vi "[Point Reactor Simulate].vi"() -> ()   [LabVIEW 2020]
doc: "本程序通过点堆动力学模型模拟核电站的反应堆运行状态。"
uses:
  <vilib>/Instr/_visa.llb/VISA Find Search Mode.ctl
  <vilib>/Utility/sysdir.llb/System Directory Type.ctl
  <vilib>/Utility/error.llb/DialogType.ctl
  Utility/Typedefs/KE622x -- Instrument Type.ctl
  Configure/Source/Typedefs/KE622x -- Voltage Limit.ctl
  Configure/Source/Typedefs/KE622x -- Current Range.ctl
  Configure/Source/Typedefs/KE622x -- Current Ranges.ctl
  <vilib>/DAQmx/write.llb/DAQmx Write (Counter 1D Frequency 1Chan NSamp).vi
  <vilib>/DAQmx/write.llb/DAQmx Write (Analog DBL 1Chan 1Samp).vi
  <vilib>/Analysis/polynomials.llb/Scalar Polynomial Evaluation (DBL).vi
  <vilib>/Instr/_visa.llb/VISA Configure Serial Port (Instr).vi
  <vilib>/DAQmx/create/channels.llb/DAQmx Create Channel (CO-Pulse Generation-Frequency).vi
  <vilib>/DAQmx/configure/timing.llb/DAQmx Timing (Implicit).vi
  <vilib>/DAQmx/create/channels.llb/DAQmx Create Channel (AO-Voltage-Basic).vi
  <vilib>/DAQmx/miscellaneous.llb/DAQmx Fill In Error Info.vi
  TcpModbus_SlaveServer/MB Slave Init (poly).vi
  TcpModbus_SlaveServer/MB Globals.vi
  TcpModbus_SlaveServer/MB Slave Read Holding Registers (poly).vi
  TcpModbus_SlaveServer/MB Slave Write Input Registers (poly).vi
  PointReactorDll.dll
  <vilib>/Analysis/NI_AALPro.lvlib
  Keithley 622x.lvlib
  <resource>/objmgr/daqmx.rc
panel:
  out "KE6220_2":bool
  in  "物理参数设置":bool
  in  "endian Switch":bool
  out "反应性仪输出电压":dbl[](array[numeric])
  out "输出电压":dbl[](array[numeric])
  in  "输出电流 (A)":dbl
  in  "电压输出选择":bool
  out "中子注量率 (n/cm2·s)":dbl
  out "硼总价值 (pcm)":dbl
  out "棒总价值 (pcm)":dbl
  out "硼浓度 indicator":dbl
  in  "硼浓度 (ppm)":dbl(slide)=1.0 scale=0.0..2000.0
  out "运行时间 (s)":dbl
  in  "TCP端口号":u16=502 min=1 max=9999
  out "堆芯反应性(硼+棒) (pcm)":dbl
  out "keff":dbl
  in  "S棒组":dbl(slide)=100.0 min=0.0 max=225.0 scale=0.0..225.0
  in  "A棒组":dbl(slide)=100.0 min=0.0 max=225.0 scale=0.0..225.0
  in  "B棒组":dbl(slide)=100.0 min=0.0 max=225.0 scale=0.0..225.0
  in  "C棒组":dbl(slide)=100.0 min=0.0 max=225.0 scale=0.0..225.0
  in  "堆芯后备反应性 (pcm)":dbl
  out "S棒价值":dbl
  out "A棒价值":dbl
  out "B棒价值":dbl
  out "C棒价值":dbl
  out "D棒价值":dbl
  out "中子注量曲线":dbl(graph) caption="Waveform Chart - Dark"
  in  "D棒组":dbl(slide)=100.0 min=0.0 max=225.0 scale=0.0..225.0
  out "CARD":bool
  out "KE6220_1":bool
  out "COM2":bool
  out "COM1":bool
  in  "VO 4":u16(ring)=3 items=["D棒位 (step)", "C棒位 (step)", "B棒位 (step)", "A棒位 (step)", "S棒位 (step)", "硼浓度 (ppm)", "中间量程电流 (A)", "源量程计数 (CPS)"]
  in  "VO 3":u16(ring)=2 items=["D棒位 (step)", "C棒位 (step)", "B棒位 (step)", "A棒位 (step)", "S棒位 (step)", "硼浓度 (ppm)", "中间量程电流 (A)", "源量程计数 (CPS)"]
  in  "VO 2":u16(ring)=1 items=["D棒位 (step)", "C棒位 (step)", "B棒位 (step)", "A棒位 (step)", "S棒位 (step)", "硼浓度 (ppm)", "中间量程电流 (A)", "源量程计数 (CPS)"]
  in  "VO 1":u16(ring) items=["D棒位 (step)", "C棒位 (step)", "B棒位 (step)", "A棒位 (step)", "S棒位 (step)", "硼浓度 (ppm)", "中间量程电流 (A)", "源量程计数 (CPS)"]
  in  "电信号输出设置":bool
  in  "TCP服务器开":bool
  out "Holding Registers":sgl[](array[numeric]) caption="Holding Registers (Read&Write)"
  out "Coils":bool[](array[boolean]) caption="Coils (Master can write coils)"
  in  "电流输出选择":u16(ring) items=["中间量程电流", "功率量程电流"]
  out "棒位与硼浓度":dbl[](array[numeric])
  in  "反应性控制方式":bool
  in  "归零":bool
  in  "棒速(step/min)":dbl=72.0 min=1.0 max=10000.0 step=1.0 format="%#.3g"
  in  "开始降棒":bool
  in  "降棒选择":u16(ring) items=["D棒组", "C棒组", "B棒组", "A棒组", "S棒组"]
  in  "细分时间 (ms)":u32=100 min=10 max=1000 step=1
  in  "开始":bool
  in  "时间比例尺":dbl(knob)=1.0 min=0.1 max=1000.0 step=0.1 scale=0.1..1000.0
  out "功率量程 (A)":dbl(slide) scale=2.875e-12..0.00023 scale format="%#_6e"
  out "中间量程 (A)":dbl(slide) scale=1e-11..0.0008 scale format="%#_6e"
  out "源量程 (CPS)":dbl(slide) scale=1.0..1000000.0 scale format="%#_6f"
  out "%FP":dbl(slide) scale=2e-09..200.0 scale format="%#_6e"
  out "中子注量率":dbl(slide) scale=0.1..10000000000.0 scale format="%#_6e"
  in  "时间步长 (s)":dbl=0.1
  in  "初始注量率 (n/cm2·s)":dbl=1.0
  in  "堆芯反应性 (pcm)":dbl
  in  "停止":bool
  in  "初始反应性 (pcm)":dbl
  # "反应性仪测试用点堆模拟器"
  # "探测器"
  # "手输"
  # "棒硼"
  # "1.25E+5 n/cm2·s\n——"
  # "——\n1.25E+2 n/cm2·s"
  # "——  1.25E-1 n/cm2·s"
  # "硬件测试"
  # "小端"
  # "0-10V"
  # "1-5V"
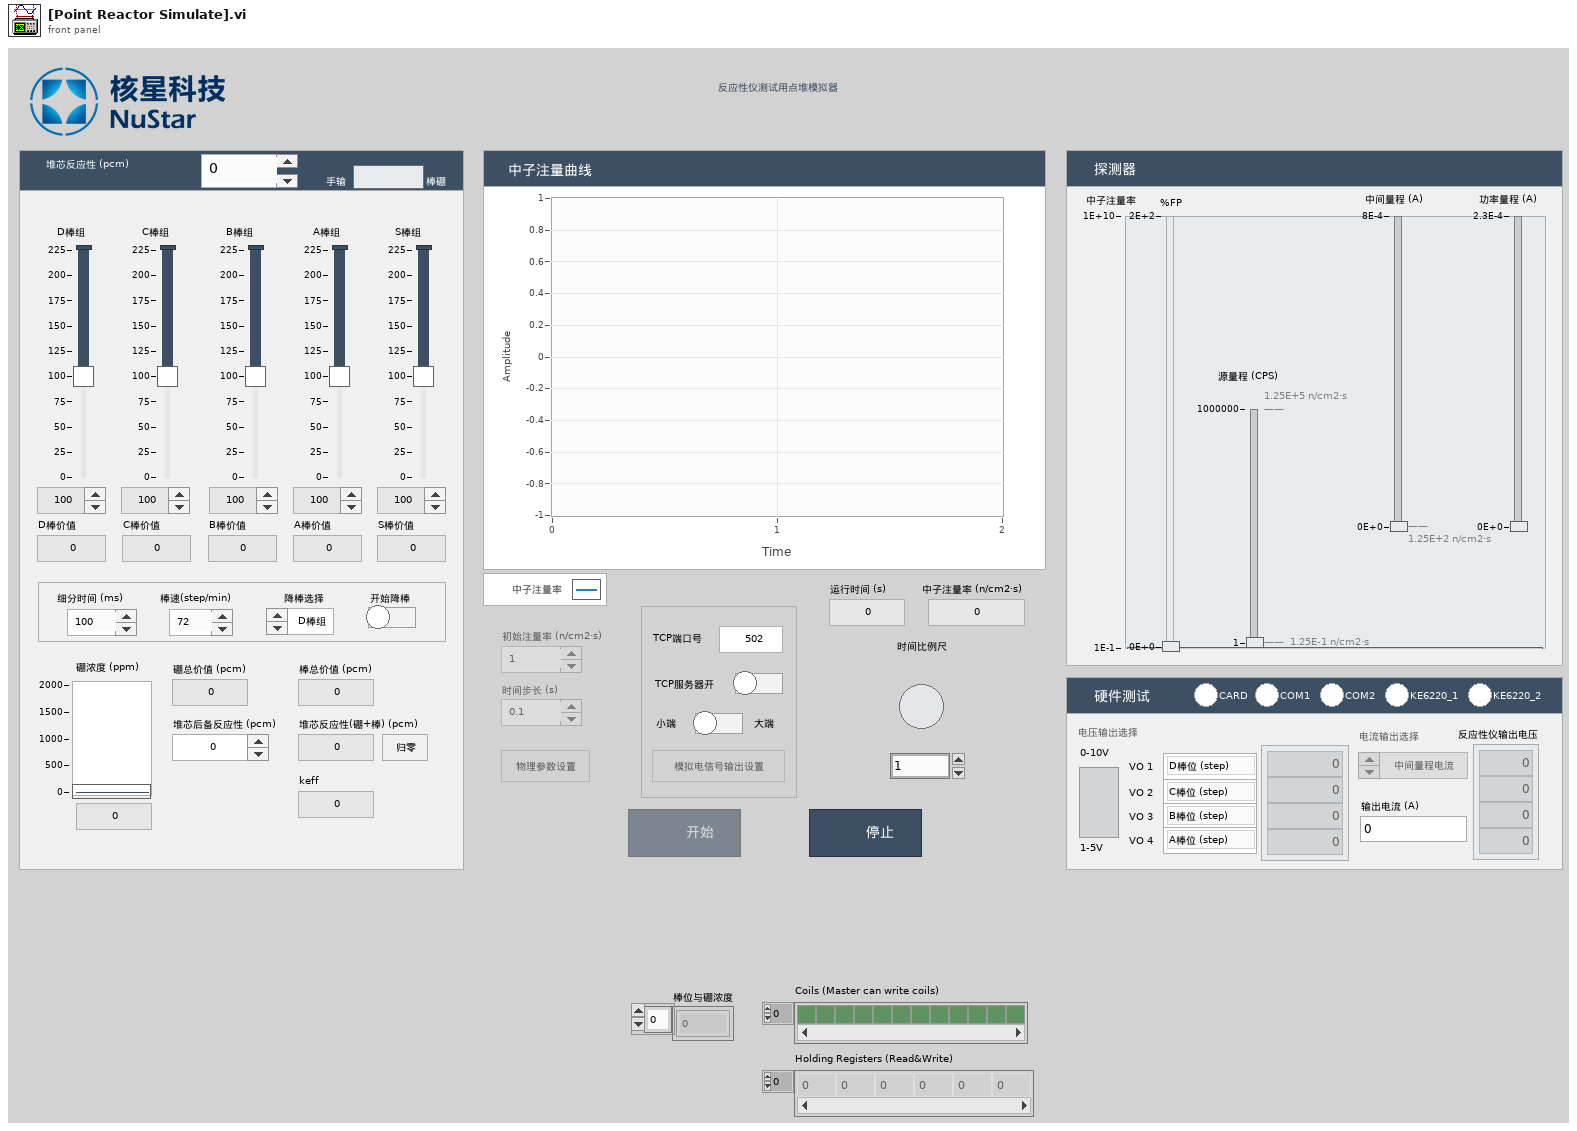
[diagram p1: front panel]
types:
  T1 = enum8{"Enabled", "Disabled", "Disabled and Grayed Out"}
  T2 = typedef "System Directory Type.ctl" = i32
  T3 = typedef "VISA Find Search Mode.ctl" = u32
  T4 = enum16{"open", "open or create", "create or replace", "create", "open (read only)"}
  T5 = typedef "DialogType.ctl" = u16
  T6 = typedef "Keithley 622x.lvlib/KE622x -- Voltage Limit.ctl" = dbl
  T7 = typedef "Keithley 622x.lvlib/KE622x -- Instrument Type.ctl" = enum16{"KE6220", "KE6221"}
  T8 = typedef "Keithley 622x.lvlib/KE622x -- Current Range.ctl" = cluster{"Auto Range?":bool, "Man / Selected\nRange":T9}
  T9 = typedef "Keithley 622x.lvlib/KE622x -- Current Ranges.ctl" = enum16{"2nA", "20nA", "200nA", "2uA", "20uA", "200uA", "2mA", "20mA", "100mA"}
  T10 = enum32{"invalid app kind", "Development System", "Run Time System", "Student Edition", "Embedded LabVIEW", "Evaluation", "Custom"}
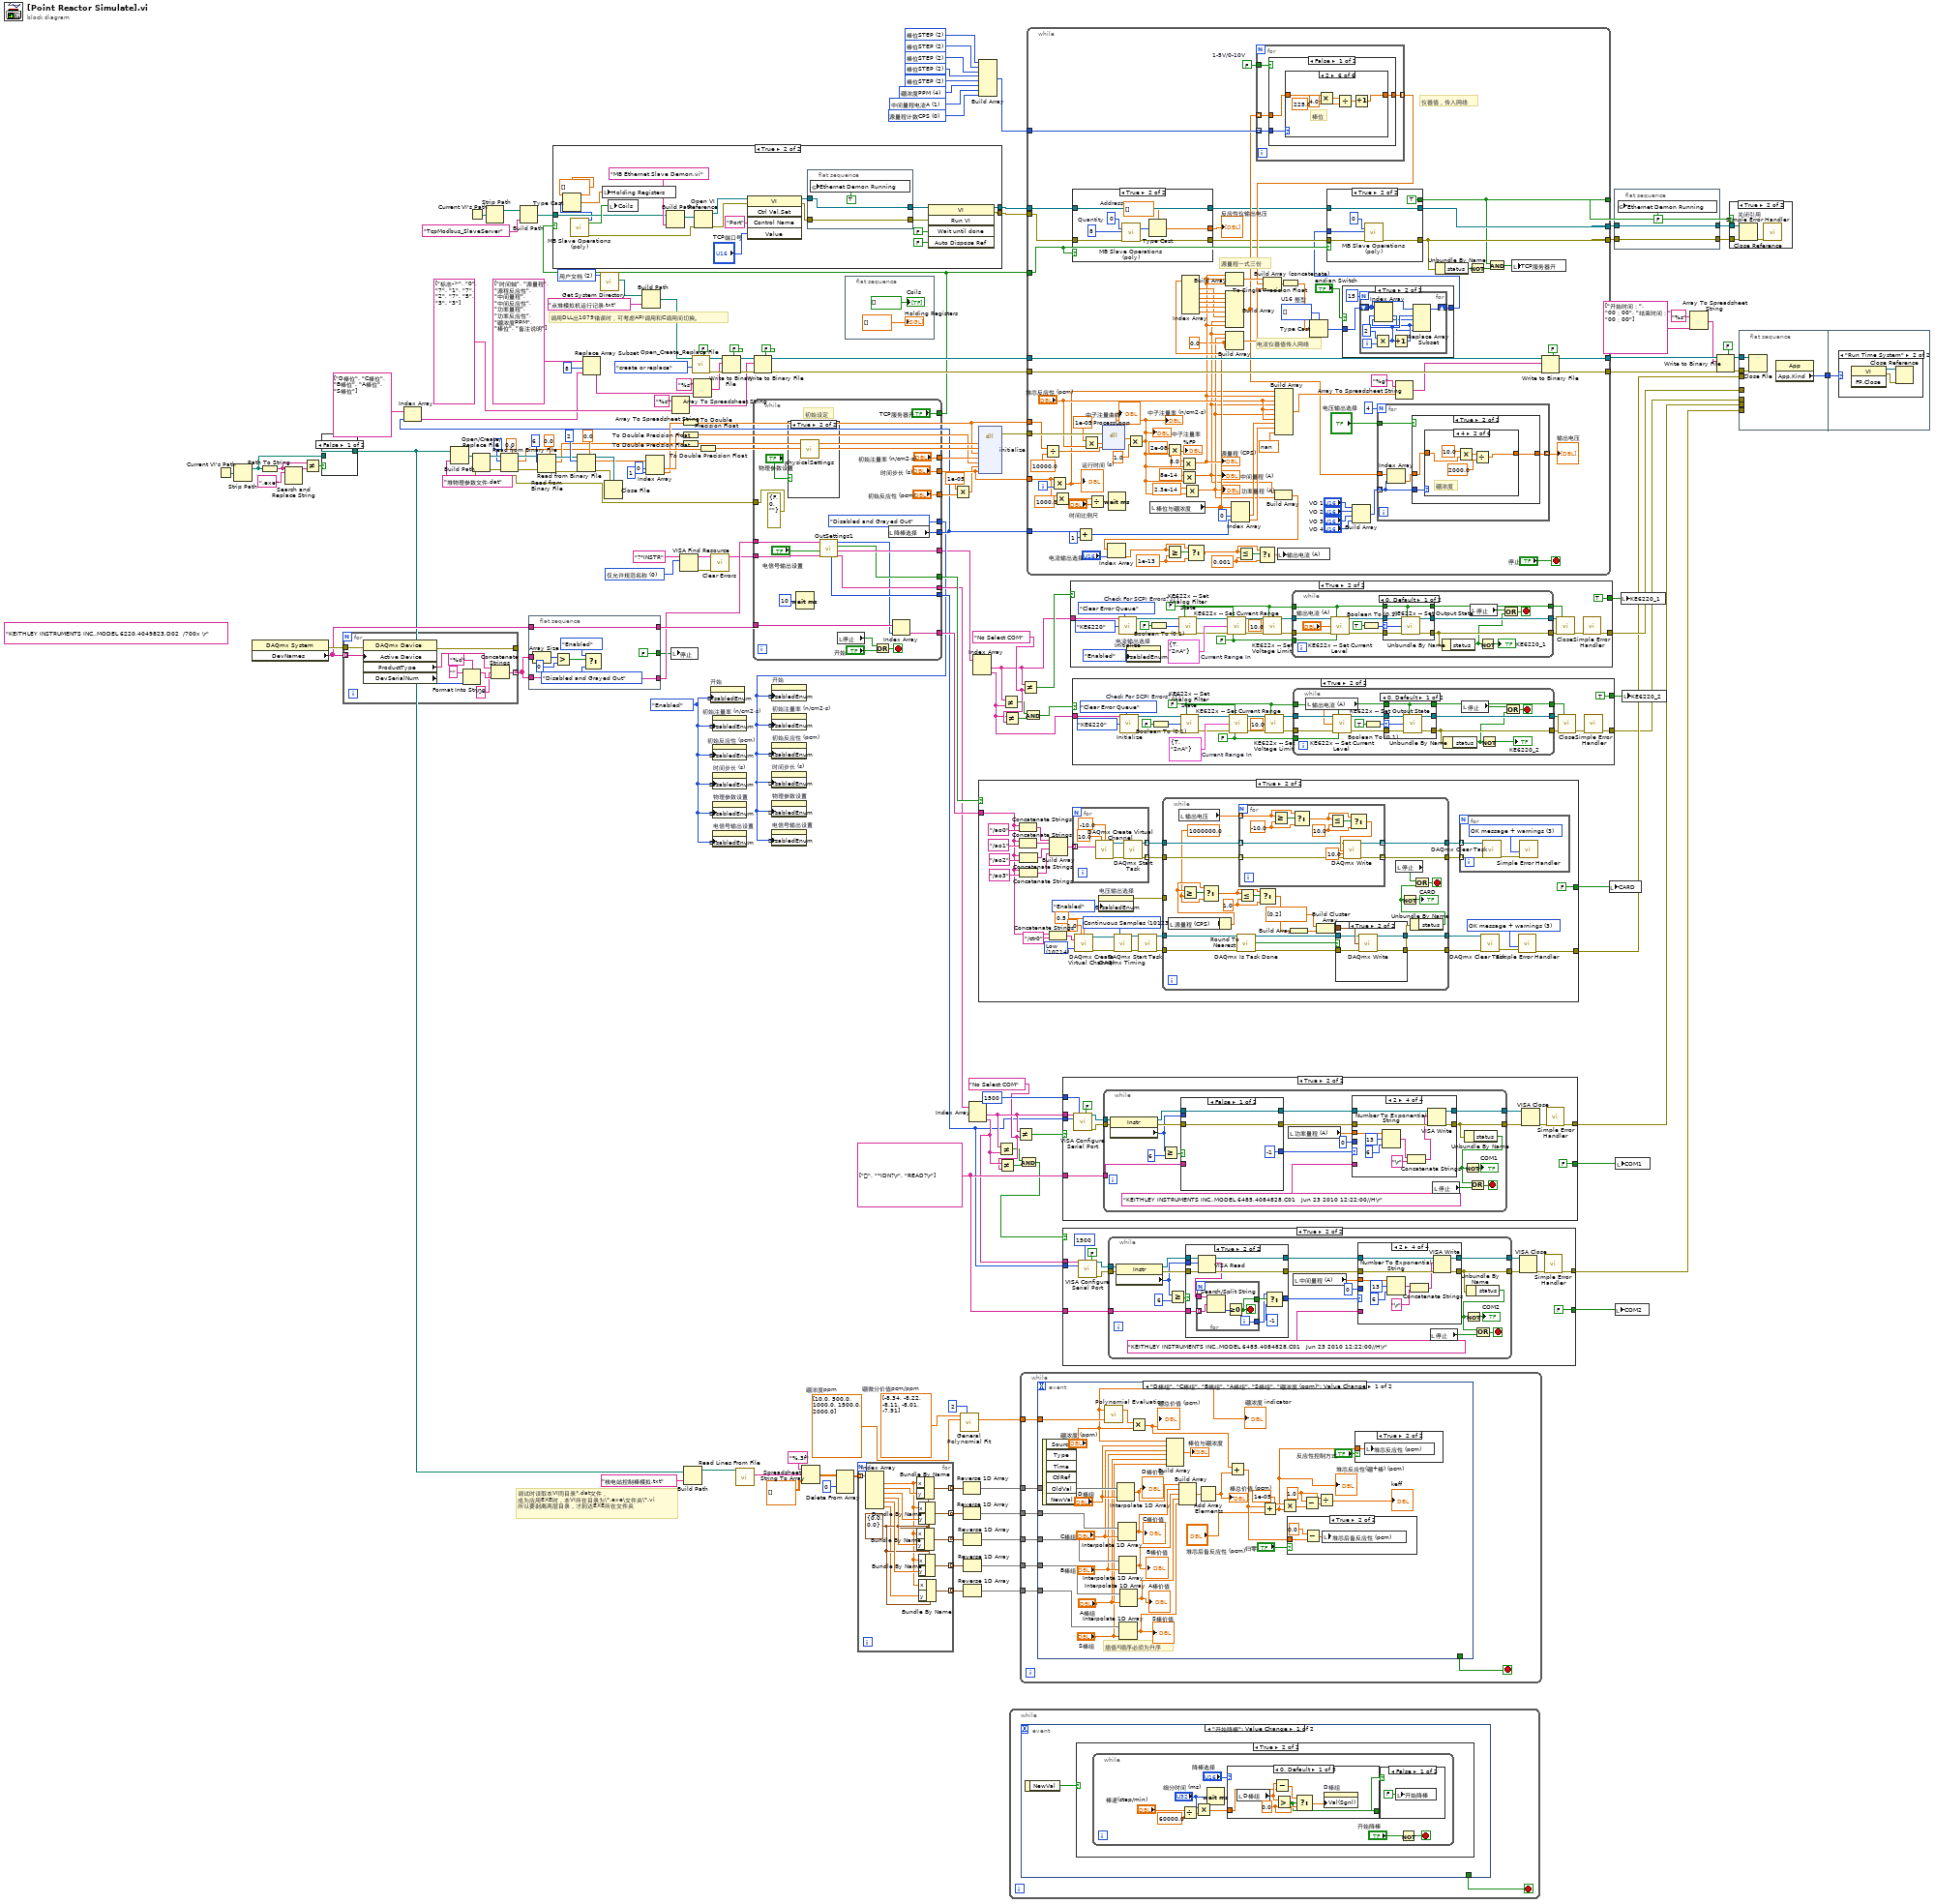
[diagram p0: block diagram]
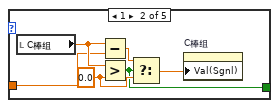
[diagram p4: hidden frame]
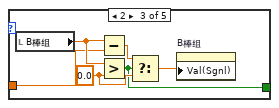
[diagram p5: hidden frame]
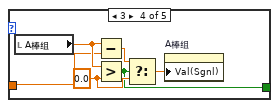
[diagram p6: hidden frame]
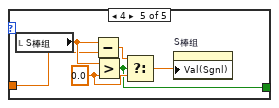
[diagram p7: hidden frame]
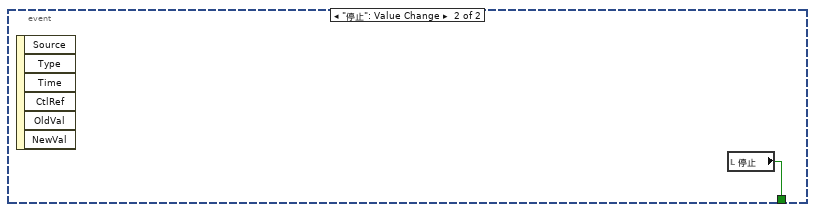
[diagram p8: hidden frame]
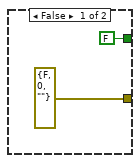
[diagram p9: hidden frame]
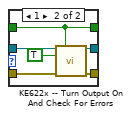
[diagram p10: hidden frame]
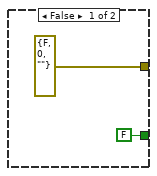
[diagram p11: hidden frame]
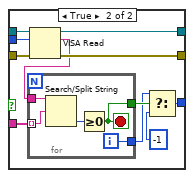
[diagram p12: hidden frame]
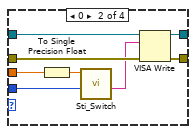
[diagram p14: hidden frame]
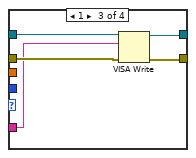
[diagram p15: hidden frame]
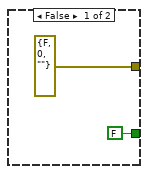
[diagram p16: hidden frame]
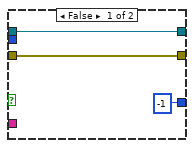
[diagram p17: hidden frame]
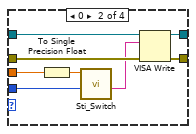
[diagram p19: hidden frame]
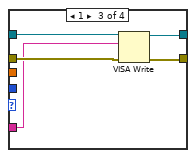
[diagram p20: hidden frame]
diagram:
  w2 = T1."Enabled" ("禁用")
  w10 = "No Select COM" ("新元素/子数组")
  (unwired) "KEITHLEY INSTRUMENTS INC.,MODEL 6220,4049823,D02  /700x \r" ("y")
  w16 = T2 2 items=["用户目录"=0, "用户桌面"=1, "用户文档"=2, "用户应用程序数据"=3, "用户设置"=4, "用户临时目录"=5, "公共文档"=6, "公共应用程序数据"=7, "公共设置"=8, "公共缓存"=13, "系统核心库"=9, "系统安装库"=10, "应用程序文件"=11, "启动盘根目录"=12] ("system directory type")
  w36 = "No Select COM" ("新元素/子数组")
  w41 = string[] ["", "*IDN?\r", "READ?\r"] ("添加的数组")
  w51 = u16 0 items=["源量程计数CPS", "中间量程电流A", "棒位STEP", "温度(摄氏度)", "硼浓度PPM", "P2电压信号"] ("P2-8")
  w50 = u16 1 items=["源量程计数CPS", "中间量程电流A", "棒位STEP", "温度(摄氏度)", "硼浓度PPM", "P2电压信号"] ("P2-7")
  w49 = u16 4 items=["源量程计数CPS", "中间量程电流A", "棒位STEP", "温度(摄氏度)", "硼浓度PPM", "P2电压信号"] ("P2-6")
  w48 = u16 2 items=["源量程计数CPS", "中间量程电流A", "棒位STEP", "温度(摄氏度)", "硼浓度PPM", "P2电压信号"] ("P2-5")
  w47 = u16 2 items=["源量程计数CPS", "中间量程电流A", "棒位STEP", "温度(摄氏度)", "硼浓度PPM", "P2电压信号"] ("P2-4")
  w46 = u16 2 items=["源量程计数CPS", "中间量程电流A", "棒位STEP", "温度(摄氏度)", "硼浓度PPM", "P2电压信号"] ("P2-3")
  w45 = u16 2 items=["源量程计数CPS", "中间量程电流A", "棒位STEP", "温度(摄氏度)", "硼浓度PPM", "P2电压信号"] ("P2-2")
  w44 = u16 2 items=["源量程计数CPS", "中间量程电流A", "棒位STEP", "温度(摄氏度)", "硼浓度PPM", "P2电压信号"] ("P2-1")
  w64 = T3 0 items=["仅允许规范名称"=0, "只允许别名"=2, "包含匹配别名"=3, "包含所有别名"=4] ("Search Mode")
  w90 = dbl[] [-8.34, -8.22, -8.11, -8.01, -7.91]  # 硼微分价值pcm/ppm
  w89 = dbl[] [10.0, 500.0, 1000.0, 1500.0, 2000.0]  # 硼浓度ppm
  # "调试时读取本VI同目录*.dat文件，\n成为应用EXE时，本VI所在目录为\\*.exe\\文件夹\\*.vi\n所以要剥离两层目录，才到达EXE所在文件夹"
  # "调用DLL出1079错误时，可考虑API调用和C调用间切换。"
  n1 = Current VI's Path() -> (path=w124:path)
  n2 = Strip Path(path=w124) -> (stripped path=w119:path)  [unwired: 1 out]
  n3 = property class="DAQmx System"() -> (error out=w70:errorcluster, "DevNames"=w68:tag[])  [unwired: 2 in, 1 out]
  n4 = Path To String(path=w119) -> (string=w121:string)
  n5 = Search and Replace String(input string=w121, search string=".exe" ("搜索字符串")) -> (result string=w122:string)  [unwired: 6 in, 3 out]
  n6 = Not Equal?(x=w121, y=w122) -> (x != y?=w120:bool)
  n7 = case shown="False" w120 {
    tunnel: w119 -> [w162 w164]
    tunnel: [w162 w163] -> w18
    frame False {
    }
    frame True {
      n8 = Strip Path(path=w164) -> (stripped path=w163:path)  [unwired: 1 out]
    }
  }
  n9 = for {
    tunnel: w68 -> [w174] mode=indexing
    tunnel: w70 -> [w173]
    tunnel: [w172] -> _
    tunnel: [w165] -> w69 mode=indexing
    n10 = property class="DAQmx Device"(error in=w173, "Active Device"=w174) -> (error out=w172:errorcluster, "ProductType"=w168:string, "DevSerialNum"=w169:u32)  [unwired: 1 in, 1 out]
    n11 = Format Into String(format string="%d" ("格式字符串"), initial string="" ("初始字符串"), w169) -> (resulting string=w167:string)  [unwired: 1 in, 1 out]
    n12 = Concatenate Strings(w168, "-" ("字符串"), w167) -> (w165:string)
  }
  n13 = Build Path(base path=w18, name or relative path="堆物理参数文件.dat") -> (appended path=w125:path)
  n14 = Current VI's Path() -> (path=w56:path)
  n15 = Strip Path(path=w56) -> (stripped path=w55:path)  [unwired: 1 out]
  n16 = Build Path ("创建路径")(base path=w55, name or relative path="TcpModbus_SlaveServer" ("搜索字符串")) -> (appended path=w54:path)
  n17 = flat-sequence {
    tunnel: w69 -> [w183]
    tunnel: [w178] -> w42
    tunnel: w69 -> [w178]
    tunnel: w68 -> [w177]
    tunnel: [w177] -> w67
    tunnel: [FALSE ("停止")] -> w27
    frame #0 {
      n18 = Array Size(array=w183) -> (size(s)=w182:i32)
      n19 = Greater?(x=w182, y=0) -> (0:w179:bool)
      n20 = Select(t=T1."Enabled" ("禁用"), s=w179, f=T1."Disabled and Grayed Out" ("禁用")) -> ()  [unwired: 1 out]
    }
  }
  n21 = call <vilib>:"Get System Directory.vi"("system directory type"=w16) -> ("system directory"=w17:path)  [unwired: 10 in]
  n22 = Build Path(base path=w17, name or relative path="点堆模拟机运行记录.txt") -> (appended path=w134:path)
  n23 = local write "停止"(w27) -> ()
  n24 = Array To Spreadsheet String(array=string[] ["标志->", "0", "7", "1", "7", "2", "7", "5", "3", "3"] ("添加的数组"), 3:"%s" ("format string")) -> (spreadsheet string=w147:string)  [unwired: 1 in]
  n25 = VISA Find Resource(10:w64, 11:"?*INSTR" ("表达式(\"?*\")")) -> (0:w57:errorcluster, 3:w13:string[])  [unwired: 1 in, 1 out]
  n26 = Build Path(base path=w18, name or relative path="核电站控制棒模拟.txt") -> (appended path=w107:path)
  n27 = call <vilib>:"Open_Create_Replace File.vi"("advisory dialog? (display:T)"=FALSE, "function (open:0)"=T4."create or replace", "file path"=w134) -> ("error out"=w154:errorcluster, "refnum"=w155:refnum<file>)  [unwired: 5 in, 2 out]
  n28 = property on="开始" class="Bool"("DisabledEnum"=w2) -> ()  [unwired: 2 in, 2 out]
  n29 = call <vilib>:"Clear Errors.vi"("error in (no error)"=w57) -> ()  [unwired: 5 in, 2 out]
  n30 = property on="初始注量率 (n/cm2·s)" class="DigNum (strict)"("DisabledEnum"=w2) -> ()  [unwired: 2 in, 2 out]
  n31 = property on="初始反应性 (pcm)" class="DigNum (strict)"("DisabledEnum"=w2) -> ()  [unwired: 2 in, 2 out]
  n32 = property on="时间步长 (s)" class="DigNum (strict)"("DisabledEnum"=w2) -> ()  [unwired: 2 in, 2 out]
  n33 = property on="物理参数设置" class="Bool"("DisabledEnum"=w2) -> ()  [unwired: 2 in, 2 out]
  n34 = property on="电信号输出设置" class="Bool"("DisabledEnum"=w2) -> ()  [unwired: 2 in, 2 out]
  n35 = call <vilib>:"Read Lines From File.vi"("file path (dialog if empty)"=w107) -> ("line string"=w104:string)  [unwired: 5 in, 3 out]
  n36 = while {
    tunnel: ["初始注量率 (n/cm2·s)"] -> w160
    tunnel: ["时间步长 (s)"] -> w159
    tunnel: ["初始反应性 (pcm)"] -> w131
    tunnel: [w199] -> w62
    tunnel: [w195] -> w7
    tunnel: [w194] -> w71
    tunnel: w67 -> [w202]
    tunnel: [w201] -> w66
    tunnel: ["TCP服务器开"] -> w59
    tunnel: w13 -> [w197]
    tunnel: [w192] -> w52
    tunnel: [w196] -> w32
    tunnel: w42 -> [w198]
    tunnel: [T1."Disabled and Grayed Out" ("禁用")] -> w14
    tunnel: [errorcluster {"status"=FALSE, "code"=0, "source"=""} ("error in")] -> w15
    stop <- w188 stop-if-true
    # "初始设定"
    n37 = case shown="True" "物理参数设置" {
      frame False {
      }
      frame True {
        n38 = call "physicalSettings.vi"() -> ()  [unwired: 1 in]
      }
    }
    n39 = Wait (ms)(milliseconds to wait=u32 10) -> ()  [unwired: 1 out]
    n40 = call "OutSettings1.vi"("所有串口"=w197, "执行:调用时显示前面板"="电信号输出设置", "电压脉冲卡选择"=w198) -> ("串口电流服务选定口"=w192:string[], "电流源串口选定"=w195:string[], "电压脉冲开关 2"=w194:bool, "电压脉冲卡选"=w191:u16, "波特率set"=w196:u32)  [unwired: 4 in]
    n41 = local read "停止"() -> (w190:bool)
    n42 = Or(x=w190, y="开始") -> (x .or. y?=w188:bool)
    n43 = local read "降棒选择"() -> (w199:u16)
    n44 = Index Array(array=w202, index=w191) -> (element=w201:tag)
  }
  n45 = Index Array(array=string[] ["D棒位", "C棒位", "B棒位", "A棒位", "S棒位"] ("添加的数组"), index=w62) -> (element=w73:string)
  n46 = Open/Create/Replace File(file path (use dialog)=w125, error in=w15) -> (refnum out=w130:refnum<file>, error out=w129:errorcluster)  [unwired: 4 in, 1 out]
  n47 = Read from Binary File(5:sgl 0.0 ("byte stream type"), 8:w129, 10:6 ("count"), 11:w130) -> (0:w115:errorcluster, 2:w81:sgl[], 3:w116:refnum<file>)  [unwired: 2 in, 1 out]
  n48 = Read from Binary File(5:sgl 0.0 ("byte stream type"), 8:w115, 10:6 ("count"), 11:w116) -> (0:w111:errorcluster, 2:w83:sgl[], 3:w112:refnum<file>)  [unwired: 2 in, 1 out]
  n49 = case shown="True" w59 {
    tunnel: [refnum<vi> refnum w215] -> w61
    tunnel: [errorcluster {"status"=FALSE, "code"=0, "source"=""} ("error out") w214] -> w60
    tunnel: w54 -> [_ w213]
    frame False {
    }
    frame True {
      n50 = call-poly "MB Slave Operations (poly).vi"() -> ("Holding Registers"=w212:u16[], "Coils"=w223:bool[], "error out"=w221:errorcluster)  [unwired: 1 in, 16 out]
      n51 = Type Cast(type=sgl[] [] ("添加的数组"), x=w212) -> (*(type *) &x=w211:sgl[])
      n52 = local write "Holding Registers"(w211) -> ()
      n53 = local write "Coils"(w223) -> ()
      n54 = Build Path ("创建路径")(base path=w213, name or relative path="MB Ethernet Slave Demon.vi") -> (appended path=w209:path)
      n55 = Open VI Reference(vi path=w209, error in (no error)=w221) -> (vi reference=w218:refnum<vi>, error out=w219:errorcluster)  [unwired: 4 out]
      n56 = invoke class="VI" method="Ctrl Val.Set"(reference=w218, error in=w219, "Control Name"="Port", "Value"="TCP端口号") -> (reference out=w226:refnum<vi>, error out=w225:errorcluster)  [unwired: 1 in, 3 out]
      n57 = flat-sequence {
        tunnel: [w230] -> w222
        tunnel: w225 -> [w230]
        tunnel: [w228] -> w224
        tunnel: w226 -> [w228]
        frame #0 {
          n58 = global write "MB Globals.vi" "Ethernet Demon Running"(TRUE ("Slave Demon Running")) -> ()
        }
      }
      n59 = invoke class="VI" method="Run VI"(reference=w224, error in=w222, "Wait until done"=FALSE, "Auto Dispose Ref"=FALSE) -> (reference out=w215:refnum<vi>, error out=w214:errorcluster)  [unwired: 1 in, 3 out]
    }
  }
  n60 = Read from Binary File(5:sgl 0.0 ("byte stream type"), 8:w111, 10:2 ("count"), 11:w112) -> (0:w109:errorcluster, 2:w86:sgl[], 3:w110:refnum<file>)  [unwired: 2 in, 1 out]
  n61 = Replace Array Subset(array=string[] ["时间轴", "源量程", "源程反应性", "中间量程", "中间反应性", "功率量程", "功率反应性", "硼浓度PPM", "棒位", "备注说明"] ("添加的数组"), new element=w73, index=8 ("索引")) -> (w72:string[])
  n62 = Close File(refnum=w110, error in=w109) -> ()  [unwired: 2 out]
  n63 = Index Array(array=w86, index #1=0 ("索引"), index #2=1 ("索引")) -> (element #1=w79:sgl, element #2=w77:sgl)
  n64 = To Double Precision Float(number=w77) -> (double precision float=w76:dbl)
  n65 = To Double Precision Float(number=w79) -> (double precision float=w78:dbl)
  n66 = To Double Precision Float(number=w83) -> (double precision float=w82:dbl[])
  n67 = Array To Spreadsheet String(array=w72, 3:"%s" ("format string")) -> (spreadsheet string=w152:string)  [unwired: 1 in]
  n68 = To Double Precision Float(number=w81) -> (double precision float=w80:dbl[])
  n69 = Write to Binary File(file (use dialog)=w155, data=w152, error in=w154, 5:FALSE ("预置数组或字符串大小？(T)")) -> (refnum out=w150:refnum<file>, error out=w149:errorcluster)  [unwired: 2 in, 1 out]
  n70 = Write to Binary File(file (use dialog)=w150, data=w147, error in=w149, 5:FALSE ("预置数组或字符串大小？(T)")) -> (refnum out=w145:refnum<file>, error out=w144:errorcluster)  [unwired: 2 in, 1 out]
  n71 = property on="开始" class="Bool"("DisabledEnum"=w14) -> ()  [unwired: 2 in, 2 out]
  n72 = property on="初始注量率 (n/cm2·s)" class="DigNum (strict)"("DisabledEnum"=w14) -> ()  [unwired: 2 in, 2 out]
  n73 = property on="初始反应性 (pcm)" class="DigNum (strict)"("DisabledEnum"=w14) -> ()  [unwired: 2 in, 2 out]
  n74 = property on="时间步长 (s)" class="DigNum (strict)"("DisabledEnum"=w14) -> ()  [unwired: 2 in, 2 out]
  n75 = property on="物理参数设置" class="Bool"("DisabledEnum"=w14) -> ()  [unwired: 2 in, 2 out]
  n76 = property on="电信号输出设置" class="Bool"("DisabledEnum"=w14) -> ()  [unwired: 2 in, 2 out]
  n77 = Spreadsheet String To Array ("电子表格字符串至数组转换")(format string="%.3f" ("format (%.3f)"), spreadsheet string=w104, array type (2D Dbl)=dbl[][] [] ("type (empty)")) -> (array=w103:dbl[][])  [unwired: 1 in]
  n78 = Delete From Array(array=w103, index (row)=0 ("索引 (行)")) -> (array with subset deleted=w101:dbl[][])  [unwired: 2 in, 1 out]
  n79 = flat-sequence {
    frame #0 {
      "Coils" <- bool[] [] ("Coils")
      "Holding Registers" <- sgl[] [] ("Holding Registers")
    }
  }
  n80 = for {
    tunnel: w101 -> [w245] mode=indexing
    tunnel: [w243] -> w100 mode=indexing
    tunnel: [w239] -> w98 mode=indexing
    tunnel: [w238] -> w97 mode=indexing
    tunnel: [w237] -> w96 mode=indexing
    tunnel: [w235] -> w92 mode=indexing
    w236 = cluster{"x":dbl, "y":dbl} {"x"=0.0, "y"=0.0} ("输入簇")
    n81 = Index Array(array=w245) -> (element #1=w233:dbl, element #2=w244:dbl, element #3=w242:dbl, element #4=w241:dbl, element #5=w240:dbl, element #6=w234:dbl)  [unwired: 6 in]
    n82 = Bundle By Name(cluster=w236, "x"=w233, "y"=w244) -> (w243:cluster{"x":dbl, "y":dbl})
    n83 = Bundle By Name(cluster=w236, "x"=w233, "y"=w241) -> (w238:cluster{"x":dbl, "y":dbl})
    n84 = Bundle By Name(cluster=w236, "x"=w233, "y"=w242) -> (w239:cluster{"x":dbl, "y":dbl})
    n85 = Bundle By Name(cluster=w236, "x"=w233, "y"=w240) -> (w237:cluster{"x":dbl, "y":dbl})
    n86 = Bundle By Name(cluster=w236, "x"=w233, "y"=w234) -> (w235:cluster{"x":dbl, "y":dbl})
  }
  n87 = Multiply(x=1e-05, y=w131) -> (x*y=w132:dbl)
  n88 = call <vilib>:"General Polynomial Fit.vi"("Y"=w90, "polynomial order"=2, "X"=w89) -> ("Polynomial Coefficients"=w87:dbl[])  [unwired: 9 in, 3 out]
  n89 = Reverse 1D Array(array=w100) -> (reversed array=w99:cluster{"x":dbl, "y":dbl}[])
  n90 = Reverse 1D Array(array=w98) -> (reversed array=w95:cluster{"x":dbl, "y":dbl}[])
  n91 = Reverse 1D Array(array=w97) -> (reversed array=w94:cluster{"x":dbl, "y":dbl}[])
  n92 = Reverse 1D Array(array=w96) -> (reversed array=w93:cluster{"x":dbl, "y":dbl}[])
  n93 = Reverse 1D Array(array=w92) -> (reversed array=w91:cluster{"x":dbl, "y":dbl}[])
  n94 = Index Array(array=w52) -> (element #1=w39:string, element #2=w37:string)  [unwired: 2 in]
  n95 = Index Array(array=w7) -> (element #1=w5:string, element #2=w3:string)  [unwired: 2 in]
  n96 = case shown="True" w71 {
    tunnel: w66 -> [_ w249]
    tunnel: [errorcluster {"status"=FALSE, "code"=0, "source"=""} ("error out") w251] -> w30
    tunnel: [FALSE ("停止") FALSE ("停止")] -> w23
    frame False {
      n97 = property on="电压输出选择" class="Bool (strict)"("DisabledEnum"=T1."Disabled and Grayed Out" ("禁用")) -> ()  [unwired: 2 in, 2 out]
    }
    frame True {
      w268 = 10214 items=["High"=10192, "Low"=10214] ("Idle State")
      w267 = 10123 items=["Finite Samples"=10178, "Continuous Samples"=10123] ("sample mode")
      w272 = T5 3 items=["no dialog", "OK message", "continue or stop message", "OK message + warnings", "continue/stop + warnings"] ("type of dialog (OK msg:1)")
      n98 = Concatenate Strings(w249, "/ao0") -> (w256:string)
      n99 = Concatenate Strings(w249, "/ao1") -> (w255:string)
      n100 = Concatenate Strings(w249, "/ao2") -> (w254:string)
      n101 = Concatenate Strings(w249, "/ao3") -> (w253:string)
      n102 = Concatenate Strings(w249, "/ctr0") -> (w260:string)
      n103 = Build Array(w256, w255, w254, w253) -> (w252:string[])
      n104 = for {
        tunnel: [w289] -> w278 mode=indexing
        tunnel: [w288] -> w277 mode=indexing
        tunnel: w252 -> [w287] mode=indexing
        n105 = call-poly <vilib>:"DAQmx Create Virtual Channel.vi"("maximum value"=10.0 ("Maximum Value"), "minimum value"=-10.0 ("Minimum Value"), "physical channels"=w287) -> ("task out"=w291:refnum<k21>, "error out"=w290:errorcluster)  [unwired: 11 in]
        n106 = call <vilib>:"DAQmx Start Task.vi"("task/channels in"=w291, "error in"=w290) -> ("task out"=w289:refnum<k21>, "error out"=w288:errorcluster)  [unwired: 12 in]
      }
      n107 = call-poly <vilib>:"DAQmx Create Virtual Channel.vi"("frequency"=1.0 ("duty cycle"), "duty cycle"=0.5, "counter"=w260, "idle state"=w268) -> ("task out"=w264:refnum<k21>, "error out"=w263:errorcluster)  [unwired: 10 in]
      n108 = property on="电压输出选择" class="Bool (strict)"("DisabledEnum"=T1."Enabled" ("禁用")) -> (error out=w275:errorcluster)  [unwired: 2 in, 1 out]
      n109 = call-poly <vilib>:"DAQmx Timing.vi"("task/channels in"=w264, "sample mode"=w267, "error in"=w263) -> ("task out"=w266:refnum<k21>, "error out"=w265:errorcluster)  [unwired: 11 in]
      n110 = call <vilib>:"DAQmx Start Task.vi"("task/channels in"=w266, "error in"=w265) -> ("task out"=w262:refnum<k21>, "error out"=w261:errorcluster)  [unwired: 12 in]
      n111 = while {
        tunnel: [w320] -> w281
        tunnel: [w319] -> w280
        tunnel: w278 -> [w318]
        tunnel: w277 -> [w317]
        tunnel: [w308] -> w274
        tunnel: [w304] -> w273
        tunnel: w262 -> [w299]
        tunnel: w275 -> [_]
        tunnel: w261 -> [w298]
        stop <- w301 stop-if-true
        w310 = 1000000.0 ("y")
        w313 = 1.0 ("y")
        n112 = local read "源量程 (CPS)"() -> (w316:dbl)
        n113 = local read "输出电压"() -> (w294:dbl[])
        n114 = Round To Nearest(number=w316) -> (nearest integer value=w311:dbl)
        n115 = Greater Or Equal?(x=w311, y=w310) -> (x >= y?=w315:bool)
        n116 = Select(t=w311, s=w315, f=w310) -> (s? t:f=w312:dbl)
        n117 = call <vilib>:"DAQmx Is Task Done.vi"("task/channels in"=w299, "error in"=w298) -> ("task out"=w297:refnum<k21>, "task done?"=w295:bool, "error out"=w296:errorcluster)  [unwired: 11 in]
        n118 = Less Or Equal?(x=w312, y=w313) -> (x <= y?=w314:bool)
        n119 = for {
          tunnel: [w338] -> w320 mode=indexing
          tunnel: [w337] -> w319 mode=indexing
          tunnel: w318 -> [w330] mode=indexing
          tunnel: w317 -> [w329] mode=indexing
          tunnel: w294 -> [w328] mode=indexing
          w333 = 10.0 ("y")
          w335 = -10.0 ("y")
          n120 = Greater Or Equal?(x=w328, y=w335) -> (x >= y?=w336:bool)
          n121 = Select(t=w328, s=w336, f=w335) -> (s? t:f=w332:dbl)
          n122 = Less Or Equal?(x=w332, y=w333) -> (x <= y?=w334:bool)
          n123 = Select(t=w332, s=w334, f=w333) -> (s? t:f=w331:dbl)
          n124 = call-poly <vilib>:"DAQmx Write.vi"("task/channels in"=w330, "data"=w331, "timeout"=10.0, "error in"=w329) -> ("task out"=w338:refnum<k21>, "error out"=w337:errorcluster)  [unwired: 9 in, 1 out]
        }
        n125 = Select(t=w312, s=w314, f=w313) -> (s? t:f=w305:dbl)
        n126 = Build Array(w305) -> (w306:dbl[])
        n127 = Build Cluster Array(dbl[] [0.2] ("数组"), w306) -> (w309:cluster{"initial delay":dbl, "y":dbl}[])
        n128 = case shown="True" w295 {
          tunnel: w309 -> [_ w327]
          tunnel: [w322 w326] -> w308
          tunnel: [w321 w325] -> w304
          tunnel: w297 -> [w322 w324]
          tunnel: w296 -> [w321 w323]
          frame False {
          }
          frame True {
            n129 = call-poly <vilib>:"DAQmx Write.vi"("task/channels in"=w324, "data"=w327, "error in"=w323) -> ("task out"=w326:refnum<k21>, "error out"=w325:errorcluster)  [unwired: 10 in, 1 out]
          }
        }
        n130 = local read "停止"() -> (w300:bool)
        n131 = Unbundle By Name(w304) -> ("status"=w302:bool)
        n132 = Not(x=w302) -> (.not. x?=→"CARD":bool)
        n133 = Or(x=w300, y=w302) -> (x .or. y?=w301:bool)
      }
      n134 = for {
        tunnel: w281 -> [w284] mode=indexing
        tunnel: w280 -> [w283] mode=indexing
        w285 = T5 3 items=["no dialog", "OK message", "continue or stop message", "OK message + warnings", "continue/stop + warnings"] ("type of dialog (OK msg:1)")
        n135 = call <vilib>:"DAQmx Clear Task.vi"("task in"=w284, "error in"=w283) -> ("error out"=w286:errorcluster)  [unwired: 13 in]
        n136 = call <vilib>:"Simple Error Handler.vi"("type of dialog (OK msg:1)"=w285, "error in (no error)"=w286) -> ()  [unwired: 3 in, 5 out]
      }
      n137 = call <vilib>:"DAQmx Clear Task.vi"("task in"=w274, "error in"=w273) -> ("error out"=w271:errorcluster)  [unwired: 13 in]
      n138 = call <vilib>:"Simple Error Handler.vi"("type of dialog (OK msg:1)"=w272, "error in (no error)"=w271) -> ("error out"=w251:errorcluster)  [unwired: 3 in, 4 out]
    }
  }
  n139 = Build Array(w44, w45, w46, w47, w48, w49, w50, w51) -> (w43:u16[])
  n140 = dll-call lib="D:/LVprojects/PointReactorSimulator/PointReactorDll.dll" fn="initialize"("lamd"=w82, "bet"=w80, "source"=w76, "n0"=w160, "nlife"=w78, "reactivity"=w132, "delt"=w159) -> (error out=w161:errorcluster)  [unwired: 3 in, 9 out]
  n141 = Not Equal?(x=w39, y=w37) -> (x != y?=w34:bool)
  n142 = Not Equal?(x=w37, y=w36) -> (x != y?=w35:bool)
  n143 = Not Equal?(x=w5, y=w3) -> (x != y?=w8:bool)
  n144 = Not Equal?(x=w3, y=w10) -> (x != y?=w9:bool)
  n145 = while {
    stop <- w340 stop-if-true
    n146 = event shown="[0] \"开始降棒\": Value Change" {
      selector: _ -> [_ _]
      dyn-events: _ -> [_ _]
      timeout: _ -> [_ _]
      tunnel: [_ w382] -> w340
      event "开始降棒": Value Change {
        n147 = event-data() -> ("NewVal"=w341:bool)  [unwired: 1 in]
        n148 = case shown="True" w341 {
          frame False {
          }
          frame True {
            n149 = while {
              stop <- w344 stop-if-true
              n150 = Divide(x="棒速(step/min)", y=60000.0) -> (x/y=w347:dbl)
              n151 = Multiply(x="细分时间 (ms)", y=w347) -> (x*y=w346:dbl)
              n152 = Wait (ms)(milliseconds to wait="细分时间 (ms)") -> ()  [unwired: 1 out]
              n153 = case shown="0, Default" "降棒选择" {
                tunnel: w346 -> [w356 w360 w366 w372 w378]
                tunnel: [w353 w359 w365 w371 w377] -> w342
                frame 0, Default {
                  w354 = 0.0 ("y")
                  n154 = local read "D棒组"() -> (w357:dbl)
                  n155 = Subtract(x=w357, y=w356) -> (x-y=w355:dbl)
                  n156 = Greater?(x=w357, y=w354) -> (0:w353:bool)
                  n157 = Select(t=w355, s=w353, f=w354) -> (s? t:f=w352:dbl)
                  n158 = property on="D棒组" class="Slide (strict)"("Val(Sgnl)"=w352) -> ()  [unwired: 2 in, 2 out]
                }
                frame 1 {
                  w362 = 0.0 ("y")
                  n159 = local read "C棒组"() -> (w361:dbl)
                  n160 = Subtract(x=w361, y=w360) -> (x-y=w363:dbl)
                  n161 = Greater?(x=w361, y=w362) -> (0:w359:bool)
                  n162 = Select(t=w363, s=w359, f=w362) -> (s? t:f=w358:dbl)
                  n163 = property on="C棒组" class="Slide (strict)"("Val(Sgnl)"=w358) -> ()  [unwired: 2 in, 2 out]
                }
                frame 2 {
                  w368 = 0.0 ("y")
                  n164 = local read "B棒组"() -> (w367:dbl)
                  n165 = Subtract(x=w367, y=w366) -> (x-y=w369:dbl)
                  n166 = Greater?(x=w367, y=w368) -> (0:w365:bool)
                  n167 = Select(t=w369, s=w365, f=w368) -> (s? t:f=w364:dbl)
                  n168 = property on="B棒组" class="Slide (strict)"("Val(Sgnl)"=w364) -> ()  [unwired: 2 in, 2 out]
                }
                frame 3 {
                  w374 = 0.0 ("y")
                  n169 = local read "A棒组"() -> (w373:dbl)
                  n170 = Subtract(x=w373, y=w372) -> (x-y=w375:dbl)
                  n171 = Greater?(x=w373, y=w374) -> (0:w371:bool)
                  n172 = Select(t=w375, s=w371, f=w374) -> (s? t:f=w370:dbl)
                  n173 = property on="A棒组" class="Slide (strict)"("Val(Sgnl)"=w370) -> ()  [unwired: 2 in, 2 out]
                }
                frame 4 {
                  w381 = 0.0 ("y")
                  n174 = local read "S棒组"() -> (w379:dbl)
                  n175 = Subtract(x=w379, y=w378) -> (x-y=w380:dbl)
                  n176 = Greater?(x=w379, y=w381) -> (0:w377:bool)
                  n177 = Select(t=w380, s=w377, f=w381) -> (s? t:f=w376:dbl)
                  n178 = property on="S棒组" class="Slide (strict)"("Val(Sgnl)"=w376) -> ()  [unwired: 2 in, 2 out]
                }
              }
              n179 = case shown="False" w342 {
                frame False {
                  n180 = local write "开始降棒"(FALSE ("开始降棒")) -> ()
                }
                frame True {
                }
              }
              n181 = Not(x="开始降棒") -> (.not. x?=w344:bool)
            }
          }
        }
      }
      event "停止": Value Change {
        n182 = event-data() -> ()  [unwired: 1 in, 6 out]
        n183 = local read "停止"() -> (w382:bool)
      }
    }
  }
  n184 = Not Equal?(x=w39, y=w36) -> (x != y?=w38:bool)
  n185 = And(x=w34, y=w35) -> (x .and. y?=w33:bool)
  n186 = while {
    tunnel: w99 -> [w389]
    tunnel: w95 -> [w388]
    tunnel: w94 -> [w387]
    tunnel: w93 -> [w386]
    tunnel: w91 -> [w385]
    tunnel: w87 -> [w384]
    stop <- w383 stop-if-true
    n187 = event shown="[0] \"D棒组\", \"C棒组\", \"B棒组\", \"A棒组\", \"S棒组\", \"硼浓度 (ppm)\": Value Change" {
      selector: _ -> [_ _]
      dyn-events: _ -> [_ _]
      timeout: _ -> [_ _]
      tunnel: w389 -> [w421 _]
      tunnel: w388 -> [w420 _]
      tunnel: w387 -> [w419 _]
      tunnel: w386 -> [w418 _]
      tunnel: w385 -> [w412 _]
      tunnel: w384 -> [w410 _]
      tunnel: [_ w426] -> w383
      event "D棒组", "C棒组", "B棒组", "A棒组", "S棒组", "硼浓度 (ppm)": Value Change {
        w411 = 1.0 ("x")
        # "插值X顺序必须为升序"
        n188 = event-data() -> ()  [unwired: 1 in, 6 out]
        n189 = call-poly <vilib>:"Polynomial Evaluation.vi"("P(x)"=w410, "a"="硼浓度 (ppm)") -> ("P(a)"=w409:dbl)  [unwired: 1 out]
        n190 = Interpolate 1D Array(1:"D棒组", 2:w421) -> (0:w405:dbl)
        "D棒价值" <- w405
        n191 = Interpolate 1D Array(1:"C棒组", 2:w420) -> (0:w404:dbl)
        "C棒价值" <- w404
        n192 = Interpolate 1D Array(1:"B棒组", 2:w419) -> (0:w403:dbl)
        "B棒价值" <- w403
        n193 = Interpolate 1D Array ("一维数组插值")(1:"S棒组", 2:w412) -> (0:w401:dbl)
        "S棒价值" <- w401
        n194 = Interpolate 1D Array(1:"A棒组", 2:w418) -> (0:w402:dbl)
        "A棒价值" <- w402
        n195 = Multiply(x=w409, y="硼浓度 (ppm)") -> (x*y=w390:dbl)
        "硼总价值 (pcm)" <- w390
        n196 = Build Array("硼浓度 (ppm)", "D棒组", "C棒组", "B棒组", "A棒组", "S棒组") -> (→"棒位与硼浓度":dbl[])
        n197 = Build Array(w405, w404, w403, w402, w401) -> (w417:dbl[])
        n198 = Add Array Elements(numeric array=w417) -> (sum=w391:dbl)
        "棒总价值 (pcm)" <- w391
        n199 = Add(x=w390, y=w391) -> (x+y=w406:dbl)
        n200 = Add(x=w406, y="堆芯后备反应性 (pcm)") -> (x+y=w393:dbl)
        "堆芯反应性(硼+棒) (pcm)" <- w393
        n201 = Multiply(x=1e-05, y=w393) -> (x*y=w415:dbl)
        n202 = case shown="True" "归零" {
          tunnel: w406 -> [_ w425]
          frame False {
          }
          frame True {
            n203 = Subtract(x=0.0, y=w425) -> (x-y=w424:dbl)
            n204 = local write "堆芯后备反应性 (pcm)"(w424) -> ()
          }
        }
        n205 = Subtract(x=w411, y=w415) -> (x-y=w414:dbl)
        n206 = Divide(x=w411, y=w414) -> (x/y=→"keff":dbl)
        n207 = case shown="True" "反应性控制方式" {
          tunnel: w393 -> [_ w422]
          frame False {
          }
          frame True {
            n208 = local write "堆芯反应性 (pcm)"(w422) -> ()
          }
        }
        "硼浓度 indicator" <- "硼浓度 (ppm)"
      }
      event "停止": Value Change {
        n209 = event-data() -> ()  [unwired: 1 in, 6 out]
        n210 = local read "停止"() -> (w426:bool)
      }
    }
  }
  n211 = Not Equal?(x=w5, y=w10) -> (x != y?=w6:bool)
  n212 = And(x=w8, y=w9) -> (x .and. y?=w4:bool)
  n213 = while {
    tunnel: w161 -> [w515]
    tunnel: w159 -> [w492]
    tunnel: w145 -> [w511]
    tunnel: w144 -> [w510]
    tunnel: [w509] -> w139
    tunnel: [w508] -> w140
    tunnel: w76 -> [w491]
    tunnel: w62 -> [w487]
    tunnel: w61 -> [w443]
    tunnel: w60 -> [w444]
    tunnel: [w464] -> w21
    tunnel: [w449] -> w22
    tunnel: w59 -> [w440]
    tunnel: [w446] -> w58
    tunnel: w43 -> [w462]
    i -> [w514]
    stop <- "停止" stop-if-true
    w436 = u16[] []  # U16 整型
    w438 = 0.0 ("元素")
    w463 = FALSE  # 1-5V/0-10V
    w479 = 0.001 ("y")
    w482 = 1e-13 ("y")
    # "电流仪器值传入网络"
    # "仪器值，传入网络"
    # "源量程一式三份"
    n214 = Divide(x=w491, y=10000.0) -> (x/y=w490:dbl)
    n215 = Multiply(x=w492, y=w514) -> (x*y=w432:dbl)
    "运行时间 (s)" <- w432
    n216 = Multiply(x=w492, y=1000.0) -> (x*y=w494:dbl)
    n217 = case shown="True" w440 {
      tunnel: w444 -> [w530 w538]
      tunnel: [w530 w537] -> w441
      tunnel: w443 -> [w531 w536]
      tunnel: [w531 w536] -> w442
      tunnel: [sgl[] [] ("单精度浮点") w532] -> w429
      frame False {
      }
      frame True {
        w535 = u16 8  # Quantity
        w539 = u16 0  # Address
        n218 = call-poly "MB Slave Operations (poly).vi"("Starting Address"=w539, "Quantity"=w535, "error in"=w538) -> ("Holding Registers"=w534:u16[], "error out"=w537:errorcluster)  [unwired: 1 in, 14 out]
        n219 = Type Cast(type=sgl[] [] ("单精度浮点"), x=w534) -> (*(type *) &x=w532:sgl[])
      }
    }
    "反应性仪输出电压" <- w429
    n220 = Add(x=w487, y=u16 1) -> (x+y=w473:u16)
    n221 = Multiply(x=1e-05, y="堆芯反应性 (pcm)") -> (x*y=w505:dbl)
    n222 = Divide(x=w494, y="时间比例尺") -> (x/y=w496:dbl)
    n223 = dll-call lib="D:/LVprojects/PointReactorSimulator/PointReactorDll.dll" fn="ProcessLoop"(error in=w515, "reactivity"=w505, "nmin"=w490) -> ("nflux"=w498:dbl)  [unwired: 2 in, 4 out]
    n224 = Wait (ms)(milliseconds to wait=w496) -> ()  [unwired: 1 out]
    n225 = Multiply(x=w498, y=1.0) -> (x*y=w431:dbl)
    "中子注量率" <- w431
    "中子注量曲线" <- w431
    "中子注量率 (n/cm2·s)" <- w431
    n226 = local read "棒位与硼浓度"() -> (w472:dbl[])
    n227 = Multiply(x=2e-08 ("y"), y=w431) -> (x*y=→"%FP":dbl)
    n228 = Multiply(x=8.0 ("y"), y=w431) -> (x*y=w461:dbl)
    "源量程 (CPS)" <- w461
    n229 = Multiply(x=8e-14 ("y"), y=w431) -> (x*y=w433:dbl)
    "中间量程 (A)" <- w433
    n230 = Index Array(array=w472) -> (element #1=w466:dbl, element #2=w471:dbl, element #3=w470:dbl, element #4=w469:dbl, element #5=w468:dbl, element #6=w467:dbl)  [unwired: 6 in]
    n231 = Multiply(x=2.3e-14 ("y"), y=w431) -> (x*y=w434:dbl)
    "功率量程 (A)" <- w434
    n232 = Build Array(w461, w461, w461) -> (w460:dbl[])
    n233 = Build Array(w471, w470, w469, w468, w467, w466, w433, w461) -> (w456:dbl[])
    n234 = Build Array(w433, w434, w438, w438) -> (w458:dbl[])
    n235 = Index Array(array=w472, index #1=0 ("索引"), index #2=w473) -> (element #1=w476:dbl, element #2=w475:dbl)
    n236 = for {
      tunnel: w456 -> [w635] mode=indexing
      tunnel: [w634] -> w459 mode=indexing
      tunnel: w463 -> [w636]
      tunnel: w462 -> [w633] mode=indexing
      n237 = case shown="False" w636 {
        tunnel: w635 -> [w639 w678]
        tunnel: [w638 w677] -> w634
        tunnel: w633 -> [w637 w676]
        frame False {
          n238 = case shown="2" w637 {
            tunnel: w639 -> [w642 w649 w655 w658 w665 w672]
            tunnel: [w640 w648 w655 w656 w663 w670] -> w638
            frame 3 {
              # "温度"
              n239 = Subtract(x=w642, y=275.0) -> (x-y=w643:dbl)
              n240 = Multiply(x=w643, y=4.0) -> (x*y=w645:dbl)
              n241 = Divide(x=w645, y=60.0) -> (x/y=w641:dbl)
              n242 = Increment(x=w641) -> (x+1=w640:dbl)
            }
            frame 4 {
              # "硼浓度"
              n243 = Multiply(x=4.0, y=w649) -> (x*y=w651:dbl)
              n244 = Divide(x=w651, y=2000.0) -> (x/y=w653:dbl)
              n245 = Add(x=w653, y=1.0) -> (x+y=w648:dbl)
            }
            frame Default {
            }
            frame 0 {
              # "源量程脉冲"
              n246 = Logarithm Base 10(1:w658) -> (0:w659:dbl)
              n247 = Multiply(x=w659, y=4.0) -> (x*y=w662:dbl)
              n248 = Divide(x=w662, y=7.0) -> (x/y=w657:dbl)
              n249 = Increment(x=w657) -> (x+1=w656:dbl)
            }
            frame 1 {
              # "中间量程电流"
              n250 = Logarithm Base 10(1:w665) -> (0:w666:dbl)
              n251 = Add(x=w666, y=11.0) -> (x+y=w669:dbl)
              n252 = Divide(x=w669, y=2.0) -> (x/y=w664:dbl)
              n253 = Increment(x=w664) -> (x+1=w663:dbl)
            }
            frame 2 {
              # "棒位"
              n254 = Multiply(x=w672, y=4.0) -> (x*y=w674:dbl)
              n255 = Divide(x=w674, y=225.0) -> (x/y=w671:dbl)
              n256 = Increment(x=w671) -> (x+1=w670:dbl)
            }
          }
        }
        frame True {
          n257 = case shown="2" w676 {
            tunnel: w678 -> [w680 w687 w691 w693 w699 w705]
            tunnel: [w679 w686 w691 w692 w698 w704] -> w677
            frame 3 {
              # "温度"
              n258 = Subtract(x=w680, y=275.0) -> (x-y=w681:dbl)
              n259 = Multiply(x=w681, y=10.0) -> (x*y=w683:dbl)
              n260 = Divide(x=w683, y=60.0) -> (x/y=w679:dbl)
            }
            frame 4 {
              # "硼浓度"
              n261 = Multiply(x=10.0, y=w687) -> (x*y=w689:dbl)
              n262 = Divide(x=w689, y=2000.0) -> (x/y=w686:dbl)
            }
            frame Default {
            }
            frame 0 {
              # "源量程脉冲"
              n263 = Logarithm Base 10(1:w693) -> (0:w694:dbl)
              n264 = Multiply(x=w694, y=10.0) -> (x*y=w697:dbl)
              n265 = Divide(x=w697, y=7.0) -> (x/y=w692:dbl)
            }
            frame 1 {
              # "中间量程电流"
              n266 = Logarithm Base 10(1:w699) -> (0:w700:dbl)
              n267 = Add(x=w700, y=11.0) -> (x+y=w703:dbl)
              n268 = Divide(x=w703, y=0.8) -> (x/y=w698:dbl)
            }
            frame 2 {
              # "棒位"
              n269 = Multiply(x=w705, y=10.0) -> (x*y=w707:dbl)
              n270 = Divide(x=w707, y=235.0) -> (x/y=w704:dbl)
            }
          }
        }
      }
    }
    n271 = Build Array (concatenate)(w460, w459, w458) -> (w457:dbl[])
    n272 = Build Array(w433, w434) -> (w485:dbl[])
    n273 = Index Array(array=w485, index="电流输出选择") -> (element=w481:dbl)
    n274 = Greater Or Equal?(x=w481, y=w482) -> (x >= y?=w483:bool)
    n275 = Select(t=w481, s=w483, f=w482) -> (s? t:f=w478:dbl)
    n276 = Less Or Equal?(x=w478, y=w479) -> (x <= y?=w480:bool)
    n277 = Select(t=w478, s=w480, f=w479) -> (s? t:f=w477:dbl)
    n278 = Build Array(w432, w461, "堆芯反应性 (pcm)", w433, "堆芯反应性 (pcm)", w434, "堆芯反应性 (pcm)", w476, w475, nan ("元素")) -> (w507:dbl[])
    n279 = local write "输出电流 (A)"(w477) -> ()
    n280 = To Single Precision Float(number=w457) -> (single precision float=w439:sgl[])
    n281 = Type Cast(type=w436, x=w439) -> (*(type *) &x=w437:u16[])
    n282 = case shown="True" "endian Switch" {
      tunnel: w437 -> [w517 w520]
      tunnel: [w517 w518] -> w435
      frame False {
      }
      frame True {
        n283 = for {
          N: 15 -> [_]
          shift-right: [w521] -> w518
          shift-left: w520 -> [w526]
          i -> [w528]
          n284 = Multiply(x=2, y=w528) -> (x*y=w525:i32)
          n285 = Increment(x=w525) -> (x+1=w524:i32)
          n286 = Index Array(array=w526, index #1=w525, index #2=w524) -> (element #1=w523:u16, element #2=w522:u16)
          n287 = Replace Array Subset(array=w526, new element #1=w522, index #1=w525, new element #2=w523, index #2=w524) -> (w521:u16[])
        }
      }
    }
    n288 = case shown="True" w440 {
      tunnel: w441 -> [w710 w716]
      tunnel: [w710 w715] -> w449
      tunnel: w442 -> [w711 w714]
      tunnel: [w711 w714] -> w464
      tunnel: [FALSE TRUE] -> w446
      tunnel: w435 -> [_ w712]
      frame False {
      }
      frame True {
        n289 = call-poly "MB Slave Operations (poly).vi"("Starting Address"=u16 0 ("Address"), "Input Registers"=w712, "error in"=w716) -> ("error out"=w715:errorcluster)  [unwired: 1 in, 15 out]
      }
    }
    n290 = Build Array("VO 1", "VO 2", "VO 3", "VO 4") -> (w451:u16[])
    n291 = for {
      N: 4 -> [_]
      tunnel: w456 -> [w542]
      tunnel: [w543] -> w428 mode=indexing
      tunnel: "电压输出选择" -> [w544]
      tunnel: w451 -> [w540] mode=indexing
      n292 = Index Array(array=w542, index=w540) -> (element=w541:dbl)
      n293 = case shown="True" w544 {
        tunnel: w541 -> [w547 w602]
        tunnel: [w546 w601] -> w543
        tunnel: w540 -> [w545 w600]
        frame False {
          n294 = case shown="2" w545 {
            tunnel: w547 -> [w549 w555 w561 w564 w571 w578 w583 w589 w595]
            tunnel: [w548 w554 w561 w562 w569 w576 w582 w588 w594] -> w546
            frame 4 {
              # "棒位"
              n295 = Multiply(x=w549, y=4.0) -> (x*y=w552:dbl)
              n296 = Divide(x=w552, y=235.0) -> (x/y=w550:dbl)
              n297 = Increment(x=w550) -> (x+1=w548:dbl)
            }
            frame 5 {
              # "硼浓度"
              n298 = Multiply(x=4.0, y=w555) -> (x*y=w557:dbl)
              n299 = Divide(x=w557, y=2000.0) -> (x/y=w559:dbl)
              n300 = Add(x=w559, y=1.0) -> (x+y=w554:dbl)
            }
            frame Default {
            }
            frame 7 {
              # "源量程脉冲"
              n301 = Logarithm Base 10(1:w564) -> (0:w565:dbl)
              n302 = Multiply(x=w565, y=4.0) -> (x*y=w568:dbl)
              n303 = Divide(x=w568, y=7.0) -> (x/y=w563:dbl)
              n304 = Increment(x=w563) -> (x+1=w562:dbl)
            }
            frame 6 {
              # "中间量程电流"
              n305 = Logarithm Base 10(1:w571) -> (0:w572:dbl)
              n306 = Add(x=w572, y=11.0) -> (x+y=w575:dbl)
              n307 = Divide(x=w575, y=2.0) -> (x/y=w570:dbl)
              n308 = Increment(x=w570) -> (x+1=w569:dbl)
            }
            frame 0 {
              # "棒位"
              n309 = Multiply(x=w578, y=4.0) -> (x*y=w580:dbl)
              n310 = Divide(x=w580, y=235.0) -> (x/y=w577:dbl)
              n311 = Increment(x=w577) -> (x+1=w576:dbl)
            }
            frame 1 {
              # "棒位"
              n312 = Multiply(x=w583, y=4.0) -> (x*y=w586:dbl)
              n313 = Divide(x=w586, y=235.0) -> (x/y=w584:dbl)
              n314 = Increment(x=w584) -> (x+1=w582:dbl)
            }
            frame 2 {
              # "棒位"
              n315 = Multiply(x=w589, y=4.0) -> (x*y=w592:dbl)
              n316 = Divide(x=w592, y=235.0) -> (x/y=w590:dbl)
              n317 = Increment(x=w590) -> (x+1=w588:dbl)
            }
            frame 3 {
              # "棒位"
              n318 = Multiply(x=w595, y=4.0) -> (x*y=w598:dbl)
              n319 = Divide(x=w598, y=235.0) -> (x/y=w596:dbl)
              n320 = Increment(x=w596) -> (x+1=w594:dbl)
            }
          }
        }
        frame True {
          n321 = case shown="4" w600 {
            tunnel: w602 -> [w604 w611 w615 w617 w623 w629]
            tunnel: [w603 w610 w615 w616 w622 w628] -> w601
            frame 3 {
              # "温度"
              n322 = Subtract(x=w604, y=275.0) -> (x-y=w605:dbl)
              n323 = Multiply(x=w605, y=10.0) -> (x*y=w607:dbl)
              n324 = Divide(x=w607, y=60.0) -> (x/y=w603:dbl)
            }
            frame 4 {
              # "硼浓度"
              n325 = Multiply(x=10.0, y=w611) -> (x*y=w613:dbl)
              n326 = Divide(x=w613, y=2000.0) -> (x/y=w610:dbl)
            }
            frame Default {
            }
            frame 0 {
              # "源量程脉冲"
              n327 = Logarithm Base 10(1:w617) -> (0:w618:dbl)
              n328 = Multiply(x=w618, y=10.0) -> (x*y=w621:dbl)
              n329 = Divide(x=w621, y=7.0) -> (x/y=w616:dbl)
            }
            frame 1 {
              # "中间量程电流"
              n330 = Logarithm Base 10(1:w623) -> (0:w624:dbl)
              n331 = Add(x=w624, y=11.0) -> (x+y=w627:dbl)
              n332 = Divide(x=w627, y=0.8) -> (x/y=w622:dbl)
            }
            frame 2 {
              # "棒位"
              n333 = Multiply(x=w629, y=10.0) -> (x*y=w631:dbl)
              n334 = Divide(x=w631, y=235.0) -> (x/y=w628:dbl)
            }
          }
        }
      }
    }
    "输出电压" <- w428
    n335 = Array To Spreadsheet String(array=w507, 3:"%g" ("format string")) -> (spreadsheet string=w506:string)  [unwired: 1 in]
    n336 = Unbundle By Name(w449) -> ("status"=w448:bool)
    n337 = Not(x=w448) -> (.not. x?=w447:bool)
    n338 = And(x=w446, y=w447) -> (x .and. y?=w445:bool)
    n339 = local write "TCP服务器开"(w445) -> ()
    n340 = Write to Binary File(file (use dialog)=w511, data=w506, error in=w510, 5:FALSE ("预置数组或字符串大小？(T)")) -> (refnum out=w509:refnum<file>, error out=w508:errorcluster)  [unwired: 2 in, 1 out]
  }
  n341 = case shown="True" w38 {
    tunnel: u32 1500 ("timeout (10sec)") -> [_ w730]
    tunnel: w41 -> [_ w724]
    tunnel: w32 -> [_ w723]
    tunnel: w39 -> [_ w722]
    tunnel: [errorcluster {"status"=FALSE, "code"=0, "source"=""} ("error out") w721] -> w29
    tunnel: [FALSE ("status") FALSE ("status")] -> w26
    frame False {
    }
    frame True {
      n342 = call-poly "VISA Configure Serial Port"("VISA resource name"=w722, "timeout (10sec)"=w730, "Enable Termination\nChar (T)"=FALSE ("Termination(T)"), "baud rate (9600)"=w723) -> ("VISA resource name out"=w729:refnum<visa-resource-name>, "error out"=w728:errorcluster)  [unwired: 5 in, 5 out]
      n343 = while {
        tunnel: w729 -> [w751]
        tunnel: w728 -> [w750]
        tunnel: [w745] -> w726
        tunnel: [w739] -> w725
        tunnel: w724 -> [w744]
        stop <- w738 stop-if-true
        n344 = property class="Instr"(reference=w751, error in=w750) -> (reference out=w748:refnum<visa-resource-name>, error out=w749:errorcluster, "Serial Settings:Number of Bytes at Serial Port"=w734:u32)
        n345 = Greater Or Equal?(x=w734, y=u32 6) -> (x >= y?=w732:bool)
        n346 = case shown="False" w732 {
          tunnel: w749 -> [w753 w765]
          tunnel: w748 -> [w754 w764]
          tunnel: [w753 w763] -> w747
          tunnel: [w754 w762] -> w746
          tunnel: w744 -> [_ w760]
          tunnel: w734 -> [_ w761]
          tunnel: [-1 w756] -> w743
          frame False {
          }
          frame True {
            n347 = VISA Read(VISA resource name=w764, byte count=w761, error in (no error)=w765) -> (VISA resource name out=w762:refnum<visa-resource-name>, read buffer=w759:string, error out=w763:errorcluster)  [unwired: 1 out]
            n348 = for {
              tunnel: w760 -> [w769] mode=indexing
              tunnel: w759 -> [w770]
              tunnel: [w767] -> w757
              tunnel: [w766] -> w758
              i -> [w767]
              stop <- w766 stop-if-true
              n349 = Search/Split String(string=w770, search string/char (-)=w769) -> (offset of match=w768:i32)  [unwired: 1 in, 2 out]
              n350 = Greater Or Equal To 0?(x=w768) -> (x >= 0?=w766:bool)
            }
            n351 = Select(t=w757, s=w758, f=-1) -> (s? t:f=w756:i32)
          }
        }
        n352 = local read "功率量程 (A)"() -> (w740:dbl)
        n353 = case shown="2" w743 {
          tunnel: [w772 w780 w782 w794] -> w739
          tunnel: w746 -> [w771 w779 w785 w793]
          tunnel: w747 -> [w772 w778 w783 w792]
          tunnel: [w771 w777 w784 w795] -> w745
          tunnel: w740 -> [_ w774 _ w791]
          tunnel: 0 ("Integer32") -> [_ w773 _ _]
          tunnel: "KEITHLEY INSTRUMENTS INC.,MODEL 6485,4084828,C01   Jun 23 2010 12:22:00//H\r" ("y") -> [_ _ w781 _]
          frame -1, Default {
          }
          frame 0 {
            n354 = To Single Precision Float(number=w774) -> (single precision float=w776:sgl)
            n355 = call "Sti_Switch.vi"("Integer32"=w773, "自定义浮点32"=w776) -> ("20B_StrOut"=w775:string)  [unwired: 9 in]
            n356 = VISA Write(VISA resource name=w779, write buffer=w775, error in (no error)=w778) -> (VISA resource name out=w777:refnum<visa-resource-name>, error out=w780:errorcluster)  [unwired: 1 out]
          }
          frame 1 {
            n357 = VISA Write(VISA resource name=w785, write buffer=w781, error in (no error)=w783) -> (VISA resource name out=w784:refnum<visa-resource-name>, error out=w782:errorcluster)  [unwired: 1 out]
          }
          frame 2 {
            n358 = Number To Exponential String(number=w791, precision (6)=i16 6 ("精度(6)"), 3:i16 13 ("宽度(-)")) -> (E-format string=w788:string)  [unwired: 1 in]
            n359 = Concatenate Strings(w788, "\r" ("字符串")) -> (w787:string)
            n360 = VISA Write(VISA resource name=w793, write buffer=w787, error in (no error)=w792) -> (VISA resource name out=w795:refnum<visa-resource-name>, error out=w794:errorcluster)  [unwired: 1 out]
          }
        }
        n361 = local read "停止"() -> (w737:bool)
        n362 = Unbundle By Name(w739) -> ("status"=w736:bool)
        n363 = Not(x=w736) -> (.not. x?=→"COM1":bool)
        n364 = Or(x=w736, y=w737) -> (x .or. y?=w738:bool)
      }
      n365 = VISA Close(VISA resource name=w726, error in (no error)=w725) -> (error out=w727:errorcluster)
      n366 = call <vilib>:"Simple Error Handler.vi"("error in (no error)"=w727) -> ("error out"=w721:errorcluster)  [unwired: 1 in, 7 out]
    }
  }
  n367 = case shown="True" w33 {
    tunnel: w41 -> [_ w802]
    tunnel: w37 -> [_ w801]
    tunnel: w32 -> [_ w800]
    tunnel: [errorcluster {"status"=FALSE, "code"=0, "source"=""} ("error out") w799] -> w28
    tunnel: [FALSE ("status") FALSE ("status")] -> w25
    frame False {
    }
    frame True {
      n368 = call-poly "VISA Configure Serial Port"("VISA resource name"=w801, "timeout (10sec)"=u32 1500, "Enable Termination\nChar (T)"=FALSE ("Termination(T)"), "baud rate (9600)"=w800) -> ("VISA resource name out"=w805:refnum<visa-resource-name>, "error out"=w806:errorcluster)  [unwired: 5 in, 5 out]
      n369 = while {
        tunnel: w805 -> [w829]
        tunnel: w806 -> [w828]
        tunnel: [w823] -> w808
        tunnel: [w817] -> w809
        tunnel: w802 -> [w822]
        stop <- w816 stop-if-true
        n370 = property class="Instr"(reference=w829, error in=w828) -> (reference out=w826:refnum<visa-resource-name>, error out=w827:errorcluster, "Serial Settings:Number of Bytes at Serial Port"=w811:u32)
        n371 = Greater Or Equal?(x=w811, y=u32 6) -> (x >= y?=w810:bool)
        n372 = case shown="True" w810 {
          tunnel: w827 -> [w831 w843]
          tunnel: w826 -> [w832 w842]
          tunnel: [w831 w841] -> w825
          tunnel: [w832 w840] -> w824
          tunnel: w822 -> [_ w838]
          tunnel: w811 -> [_ w839]
          tunnel: [-1 w834] -> w821
          frame False {
          }
          frame True {
            n373 = VISA Read(VISA resource name=w842, byte count=w839, error in (no error)=w843) -> (VISA resource name out=w840:refnum<visa-resource-name>, read buffer=w837:string, error out=w841:errorcluster)  [unwired: 1 out]
            n374 = for {
              tunnel: w838 -> [w847] mode=indexing
              tunnel: w837 -> [w848]
              tunnel: [w845] -> w835
              tunnel: [w844] -> w836
              i -> [w845]
              stop <- w844 stop-if-true
              n375 = Search/Split String(string=w848, search string/char (-)=w847) -> (offset of match=w846:i32)  [unwired: 1 in, 2 out]
              n376 = Greater Or Equal To 0?(x=w846) -> (x >= 0?=w844:bool)
            }
            n377 = Select(t=w835, s=w836, f=-1) -> (s? t:f=w834:i32)
          }
        }
        n378 = local read "中间量程 (A)"() -> (w818:dbl)
        n379 = case shown="2" w821 {
          tunnel: [w850 w858 w860 w872] -> w817
          tunnel: w824 -> [w849 w857 w863 w871]
          tunnel: w825 -> [w850 w856 w861 w870]
          tunnel: [w849 w855 w862 w873] -> w823
          tunnel: w818 -> [_ w852 _ w869]
          tunnel: 0 ("Integer32") -> [_ w851 _ _]
          tunnel: "KEITHLEY INSTRUMENTS INC.,MODEL 6485,4084828,C01   Jun 23 2010 12:22:00//H\r" ("y") -> [_ _ w859 _]
          frame -1, Default {
          }
          frame 0 {
            n380 = To Single Precision Float(number=w852) -> (single precision float=w854:sgl)
            n381 = call "Sti_Switch.vi"("Integer32"=w851, "自定义浮点32"=w854) -> ("20B_StrOut"=w853:string)  [unwired: 9 in]
            n382 = VISA Write(VISA resource name=w857, write buffer=w853, error in (no error)=w856) -> (VISA resource name out=w855:refnum<visa-resource-name>, error out=w858:errorcluster)  [unwired: 1 out]
          }
          frame 1 {
            n383 = VISA Write(VISA resource name=w863, write buffer=w859, error in (no error)=w861) -> (VISA resource name out=w862:refnum<visa-resource-name>, error out=w860:errorcluster)  [unwired: 1 out]
          }
          frame 2 {
            n384 = Number To Exponential String(number=w869, precision (6)=i16 6 ("精度(6)"), 3:i16 13 ("宽度(-)")) -> (E-format string=w866:string)  [unwired: 1 in]
            n385 = Concatenate Strings(w866, "\r" ("字符串")) -> (w865:string)
            n386 = VISA Write(VISA resource name=w871, write buffer=w865, error in (no error)=w870) -> (VISA resource name out=w873:refnum<visa-resource-name>, error out=w872:errorcluster)  [unwired: 1 out]
          }
        }
        n387 = local read "停止"() -> (w815:bool)
        n388 = Unbundle By Name(w817) -> ("status"=w813:bool)
        n389 = Not(x=w813) -> (.not. x?=→"COM2":bool)
        n390 = Or(x=w813, y=w815) -> (x .or. y?=w816:bool)
      }
      n391 = VISA Close(VISA resource name=w808, error in (no error)=w809) -> (error out=w807:errorcluster)
      n392 = call <vilib>:"Simple Error Handler.vi"("error in (no error)"=w807) -> ("error out"=w799:errorcluster)  [unwired: 1 in, 7 out]
    }
  }
  n393 = case shown="True" w6 {
    tunnel: w5 -> [_ w900]
    tunnel: [errorcluster {"status"=FALSE, "code"=0, "source"=""} ("error out") w878] -> w31
    tunnel: [FALSE ("停止") TRUE ("停止")] -> w24
    frame False {
      n394 = property on="电流输出选择" class="Ring (strict)"("DisabledEnum"=T1."Disabled and Grayed Out" ("禁用")) -> ()  [unwired: 2 in, 2 out]
    }
    frame True {
      w892 = T8 {"Auto Range?"=TRUE, "Man / Selected\nRange"=enum."2nA"}  # Current Range In
      w899 = FALSE  # Check For SCPI Errors? (T)
      w896 = FALSE ("Read Back Set Values? (T)")
      n395 = call "Initialize.vi"("VISA resource name"=w900, "Error Queue Option"=enum16{"Clear Error Queue", "Error Query"}."Clear Error Queue", "Instrument Type"=KE622x_--_Instrument_Type."KE6220") -> ("VISA resource name out"=w890:refnum<visa-resource-name>, "error out"=w889:errorcluster)  [unwired: 11 in]
      n396 = property on="电流输出选择" class="Ring (strict)"("DisabledEnum"=T1."Enabled" ("禁用")) -> ()  [unwired: 2 in, 2 out]
      n397 = Boolean To (0,1)(Boolean=FALSE ("布尔")) -> (0, 1=w882:i16)
      n398 = call "KE622x -- Set Analog Filter State.vi"("Resource In"=w890, "Check For SCPI Errors? (T)"=w899, "Analog Filter State"=w882, "error in (no error)"=w889) -> ("Resource Out (dupl)"=w886:refnum<visa-resource-name>, "error out"=w887:errorcluster)  [unwired: 10 in]
      n399 = call "KE622x -- Set Current Range.vi"("Resource In"=w886, "Check For SCPI Errors? (T)"=w899, "Current Range In"=w892, "error in (no error)"=w887, "Read Back Set Values? (T)"=w896) -> ("Resource Out (dupl)"=w884:refnum<visa-resource-name>, "error out"=w883:errorcluster)  [unwired: 8 in, 1 out]
      n400 = call "KE622x -- Set Voltage Limit.vi"("Resource In"=w884, "Check For SCPI Errors? (T)"=w899, "Voltage Limit (V)"=T6 10.0, "error in (no error)"=w883) -> ("Resource Out (dupl)"=w898:refnum<visa-resource-name>, "error out"=w897:errorcluster)  [unwired: 10 in]
      n401 = while {
        tunnel: w899 -> [w916]
        tunnel: w898 -> [w915]
        tunnel: w897 -> [w914]
        tunnel: w896 -> [w913]
        tunnel: [w912] -> w895
        tunnel: [w911] -> w894
        tunnel: [w906] -> w893
        stop <- w903 stop-if-true
        n402 = call "KE622x -- Set Current Level.vi"("Resource In"=w915, "Check For SCPI Errors? (T)"=w916, "Current Level (A) In"="输出电流 (A)", "error in (no error)"=w914, "Read Back Set Value? (T)"=w913) -> ("Resource Out (dupl)"=w910:refnum<visa-resource-name>, "error out"=w909:errorcluster)  [unwired: 8 in, 1 out]
        n403 = Boolean To (0,1)(Boolean=TRUE ("布尔")) -> (0, 1=w908:i16)
        n404 = case shown="0, Default" w908 {
          selector: w908 -> [w920 _]
          tunnel: w910 -> [w922 w928]
          tunnel: w909 -> [w921 w927]
          tunnel: [w919 w925] -> w906
          tunnel: w916 -> [w917 w923]
          tunnel: [w918 w924] -> w911
          tunnel: [w917 w923] -> w912
          frame 0, Default {
            n405 = call "KE622x -- Set Output State.vi"("Resource In"=w922, "Check For SCPI Errors? (T)"=w917, "Output State"=w920, "error in (no error)"=w921) -> ("Resource Out (dupl)"=w918:refnum<visa-resource-name>, "error out"=w919:errorcluster)  [unwired: 10 in]
          }
          frame 1 {
            n406 = call "KE622x -- Turn Output On And Check For Errors.vi"("Resource In"=w928, "Check For SCPI Errors? (T)"=w923, "Turn Off Output If Compliance?"=TRUE ("Turn Off Output\nIf Voltage Limit?"), "error in (no error)"=w927) -> ("Resource Out (dupl)"=w924:refnum<visa-resource-name>, "error out"=w925:errorcluster)  [unwired: 8 in, 2 out]
          }
        }
        n407 = Unbundle By Name(w906) -> ("status"=w902:bool)
        n408 = local read "停止"() -> (w904:bool)
        n409 = Not(x=w902) -> (.not. x?=→"KE6220_1":bool)
        n410 = Or(x=w904, y=w902) -> (x .or. y?=w903:bool)
      }
      n411 = call "Close.vi"("VISA resource name"=w894, "Query For SCPI Errors? (T)"=w895, "error in (no error)"=w893) -> ("error out"=w880:errorcluster)  [unwired: 12 in]
      n412 = call <vilib>:"Simple Error Handler.vi"("error in (no error)"=w880) -> ("error out"=w878:errorcluster)  [unwired: 4 in, 4 out]
    }
  }
  n413 = case shown="True" w4 {
    tunnel: w3 -> [_ w953]
    tunnel: [errorcluster {"status"=FALSE, "code"=0, "source"=""} ("error out") w932] -> w11
    tunnel: [FALSE ("停止") TRUE ("停止")] -> w12
    frame False {
    }
    frame True {
      w945 = T8 {"Auto Range?"=TRUE, "Man / Selected\nRange"=enum."2nA"}  # Current Range In
      w952 = FALSE  # Check For SCPI Errors? (T)
      w949 = FALSE ("Read Back Set Values? (T)")
      n414 = call "Initialize.vi"("VISA resource name"=w953, "Error Queue Option"=enum16{"Clear Error Queue", "Error Query"}."Clear Error Queue", "Instrument Type"=KE622x_--_Instrument_Type."KE6220") -> ("VISA resource name out"=w943:refnum<visa-resource-name>, "error out"=w942:errorcluster)  [unwired: 11 in]
      n415 = Boolean To (0,1)(Boolean=FALSE ("布尔")) -> (0, 1=w935:i16)
      n416 = call "KE622x -- Set Analog Filter State.vi"("Resource In"=w943, "Check For SCPI Errors? (T)"=w952, "Analog Filter State"=w935, "error in (no error)"=w942) -> ("Resource Out (dupl)"=w939:refnum<visa-resource-name>, "error out"=w940:errorcluster)  [unwired: 10 in]
      n417 = call "KE622x -- Set Current Range.vi"("Resource In"=w939, "Check For SCPI Errors? (T)"=w952, "Current Range In"=w945, "error in (no error)"=w940, "Read Back Set Values? (T)"=w949) -> ("Resource Out (dupl)"=w937:refnum<visa-resource-name>, "error out"=w936:errorcluster)  [unwired: 8 in, 1 out]
      n418 = call "KE622x -- Set Voltage Limit.vi"("Resource In"=w937, "Check For SCPI Errors? (T)"=w952, "Voltage Limit (V)"=T6 10.0, "error in (no error)"=w936) -> ("Resource Out (dupl)"=w951:refnum<visa-resource-name>, "error out"=w950:errorcluster)  [unwired: 10 in]
      n419 = while {
        tunnel: w952 -> [w969]
        tunnel: w951 -> [w968]
        tunnel: w950 -> [w967]
        tunnel: w949 -> [w966]
        tunnel: [w965] -> w948
        tunnel: [w964] -> w947
        tunnel: [w959] -> w946
        stop <- w958 stop-if-true
        n420 = local read "输出电流 (A)"() -> (w954:dbl)
        n421 = call "KE622x -- Set Current Level.vi"("Resource In"=w968, "Check For SCPI Errors? (T)"=w969, "Current Level (A) In"=w954, "error in (no error)"=w967, "Read Back Set Value? (T)"=w966) -> ("Resource Out (dupl)"=w963:refnum<visa-resource-name>, "error out"=w962:errorcluster)  [unwired: 8 in, 1 out]
        n422 = Boolean To (0,1)(Boolean=TRUE ("布尔")) -> (0, 1=w961:i16)
        n423 = case shown="0, Default" w961 {
          selector: w961 -> [w973 _]
          tunnel: w963 -> [w975 w981]
          tunnel: w962 -> [w974 w980]
          tunnel: [w972 w978] -> w959
          tunnel: w969 -> [w970 w976]
          tunnel: [w971 w977] -> w964
          tunnel: [w970 w976] -> w965
          frame 0, Default {
            n424 = call "KE622x -- Set Output State.vi"("Resource In"=w975, "Check For SCPI Errors? (T)"=w970, "Output State"=w973, "error in (no error)"=w974) -> ("Resource Out (dupl)"=w971:refnum<visa-resource-name>, "error out"=w972:errorcluster)  [unwired: 10 in]
          }
          frame 1 {
            n425 = call "KE622x -- Turn Output On And Check For Errors.vi"("Resource In"=w981, "Check For SCPI Errors? (T)"=w976, "Turn Off Output If Compliance?"=TRUE ("Turn Off Output\nIf Voltage Limit?"), "error in (no error)"=w980) -> ("Resource Out (dupl)"=w977:refnum<visa-resource-name>, "error out"=w978:errorcluster)  [unwired: 8 in, 2 out]
          }
        }
        n426 = Unbundle By Name(w959) -> ("status"=w957:bool)
        n427 = local read "停止"() -> (w956:bool)
        n428 = Not(x=w957) -> (.not. x?=→"KE6220_2":bool)
        n429 = Or(x=w956, y=w957) -> (x .or. y?=w958:bool)
      }
      n430 = call "Close.vi"("VISA resource name"=w947, "Query For SCPI Errors? (T)"=w948, "error in (no error)"=w946) -> ("error out"=w933:errorcluster)  [unwired: 12 in]
      n431 = call <vilib>:"Simple Error Handler.vi"("error in (no error)"=w933) -> ("error out"=w932:errorcluster)  [unwired: 4 in, 4 out]
    }
  }
  n432 = local write "CARD"(w23) -> ()
  n433 = flat-sequence {
    tunnel: [w984] -> w20
    tunnel: w22 -> [w984]
    tunnel: [w982] -> w19
    tunnel: w21 -> [w982]
    frame #0 {
      n434 = global write "MB Globals.vi" "Ethernet Demon Running"(FALSE ("Slave Demon Running")) -> ()
    }
  }
  n435 = local write "COM2"(w25) -> ()
  n436 = local write "COM1"(w26) -> ()
  n437 = local write "KE6220_1"(w24) -> ()
  n438 = local write "KE6220_2"(w12) -> ()
  n439 = Array To Spreadsheet String(array=string[] ["开始时间：", "00：00", "结束时间：", "00：00"] ("添加的数组"), 3:"%s" ("format string")) -> (spreadsheet string=w137:string)  [unwired: 1 in]
  n440 = Write to Binary File(file (use dialog)=w139, data=w137, error in=w140, 5:FALSE ("预置数组或字符串大小？(T)")) -> (refnum out=w143:refnum<file>, error out=w142:errorcluster)  [unwired: 2 in, 1 out]
  n441 = case shown="True" w58 {
    tunnel: w19 -> [_ w986]
    tunnel: w20 -> [_ w985]
    frame False {
    }
    frame True {
      n442 = Close Reference "关闭引用"(reference=w986, error in (no error)=w985) -> (error out=w987:errorcluster)
      n443 = call <vilib>:"Simple Error Handler.vi"("error in (no error)"=w987) -> ()  [unwired: 1 in, 8 out]
    }
  }
  n444 = flat-sequence {
    tunnel: w143 -> [w990]
    tunnel: w142 -> [w989]
    tunnel: w31 -> [_]
    tunnel: w30 -> [_]
    tunnel: w29 -> [_]
    tunnel: w28 -> [_]
    tunnel: w11 -> [_]
    tunnel: [w988] -> w1
    tunnel: w1 -> [w991]
    frame #0 {
      n445 = Close File(refnum=w990, error in=w989) -> ()  [unwired: 2 out]
      n446 = property class="App"() -> ("App.Kind"=w988:T10)  [unwired: 2 in, 2 out]
    }
    frame #1 {
      n447 = case shown="\"Run Time System\"" w991 {
        frame "Development System", Default {
        }
        frame "Run Time System" {
          n448 = invoke class="VI" method="FP.Close"() -> (reference out=w992:refnum<vi>, error out=w993:errorcluster)  [unwired: 3 in, 1 out]
          n449 = Close Reference(reference=w992, error in (no error)=w993) -> ()  [unwired: 1 out]
        }
      }
    }
  }
